vi "TrajectoryBegin.vi"(8 "error in (no error)":errorcluster) -> (0 "error out":errorcluster)   [LabVIEW 2023]
uses:
  TrajectoryGlobals.vi
  <vilib>/Rock Robotics/WPI/ThirdParty/JAS_Junk/TrajLib/Trajectory_Library.lvlib
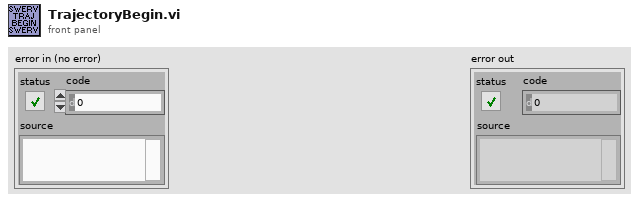
[diagram p1: front panel]
types:
  T1 = typedef "Trajectory_Library.lvlib/TRAJECTORY.ctl" = cluster{"TotalTImeSecs":dbl, "States":T2[]}
  T2 = typedef "Trajectory_Library.lvlib/TRAJ_STATE.ctl" = cluster{"TimeSeconds":dbl, "Velocity":dbl, "Acceleration":dbl, "POSE":T3, "Curvature":dbl}
  T3 = typedef "Trajectory_Library.lvlib/POSE2D.ctl" = cluster{"TRANSLATION":T4, "ROTATION":T5}
  T4 = typedef "Trajectory_Library.lvlib/TRANSLATION2D.ctl" = cluster{"X":dbl, "Y":dbl}
  T5 = typedef "Trajectory_Library.lvlib/ROTATION2D.ctl" = cluster{"VALUE":dbl, "COS":dbl, "SIN":dbl}
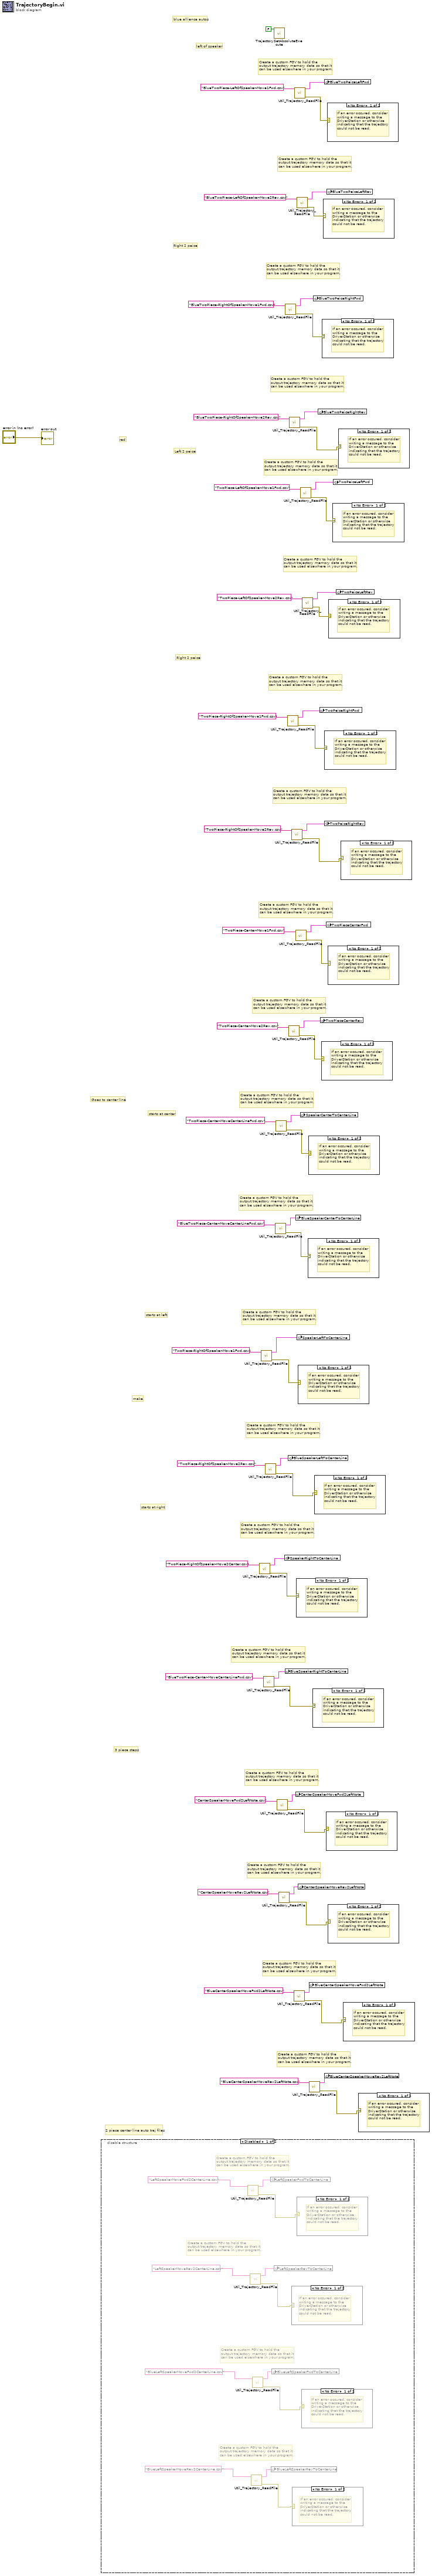
[diagram p0: block diagram]
diagram:
  # "2 piece center line auto traj files"
  # "Create a custom FGV to hold the \noutput trajectory memory data so that it\ncan be used elsewhere in your program."
  # "Create a custom FGV to hold the \noutput trajectory memory data so that it\ncan be used elsewhere in your program."
  # "Create a custom FGV to hold the \noutput trajectory memory data so that it\ncan be used elsewhere in your program."
  # "3 piece steps"
  # "Create a custom FGV to hold the \noutput trajectory memory data so that it\ncan be used elsewhere in your program."
  # "make"
  # "Create a custom FGV to hold the \noutput trajectory memory data so that it\ncan be used elsewhere in your program."
  # "Create a custom FGV to hold the \noutput trajectory memory data so that it\ncan be used elsewhere in your program."
  # "Create a custom FGV to hold the \noutput trajectory memory data so that it\ncan be used elsewhere in your program."
  # "Create a custom FGV to hold the \noutput trajectory memory data so that it\ncan be used elsewhere in your program."
  # "starts at right"
  # "starts at left"
  # "starts at center"
  # "Goes to center line"
  # "Create a custom FGV to hold the \noutput trajectory memory data so that it\ncan be used elsewhere in your program."
  # "Create a custom FGV to hold the \noutput trajectory memory data so that it\ncan be used elsewhere in your program."
  # "Create a custom FGV to hold the \noutput trajectory memory data so that it\ncan be used elsewhere in your program."
  # "Create a custom FGV to hold the \noutput trajectory memory data so that it\ncan be used elsewhere in your program."
  # "red"
  # "Right 2 peice"
  # "Create a custom FGV to hold the \noutput trajectory memory data so that it\ncan be used elsewhere in your program."
  # "Create a custom FGV to hold the \noutput trajectory memory data so that it\ncan be used elsewhere in your program."
  # "Create a custom FGV to hold the \noutput trajectory memory data so that it\ncan be used elsewhere in your program."
  # "Create a custom FGV to hold the \noutput trajectory memory data so that it\ncan be used elsewhere in your program."
  # "left of speaker"
  # "blue allience autos"
  # "Right 2 peice"
  # "Left 2 peice"
  # "Create a custom FGV to hold the \noutput trajectory memory data so that it\ncan be used elsewhere in your program."
  # "Create a custom FGV to hold the \noutput trajectory memory data so that it\ncan be used elsewhere in your program."
  # "Create a custom FGV to hold the \noutput trajectory memory data so that it\ncan be used elsewhere in your program."
  # "Create a custom FGV to hold the \noutput trajectory memory data so that it\ncan be used elsewhere in your program."
  n1 = disable-structure shown="Disabled" {
    frame Disabled {
      # "Create a custom FGV to hold the \noutput trajectory memory data so that it\ncan be used elsewhere in your program."
      # "Create a custom FGV to hold the \noutput trajectory memory data so that it\ncan be used elsewhere in your program."
      # "Create a custom FGV to hold the \noutput trajectory memory data so that it\ncan be used elsewhere in your program."
      # "Create a custom FGV to hold the \noutput trajectory memory data so that it\ncan be used elsewhere in your program."
      n2 = call <vilib>:"Util_Trajectory_ReadFile.vi"("FileName"="LeftSpeakerMoveFwd2CenterLine.csv") -> ("error out"=w72:errorcluster, "outTRAJECTORY"=w73:T1)  [unwired: 8 in, 1 out]
      n3 = call <vilib>:"Util_Trajectory_ReadFile.vi"("FileName"="LeftSpeakerMoveRev2CenterLine.csv") -> ("error out"=w69:errorcluster, "outTRAJECTORY"=w70:T1)  [unwired: 8 in, 1 out]
      n4 = call <vilib>:"Util_Trajectory_ReadFile.vi"("FileName"="BlueLeftSpeakerMoveRev2CenterLine.csv") -> ("error out"=w63:errorcluster, "outTRAJECTORY"=w64:T1)  [unwired: 8 in, 1 out]
      n5 = call <vilib>:"Util_Trajectory_ReadFile.vi"("FileName"="BlueLeftSpeakerMoveFwd2CenterLine.csv") -> ("error out"=w66:errorcluster, "outTRAJECTORY"=w67:T1)  [unwired: 8 in, 1 out]
      n6 = global write "TrajectoryGlobals.vi" "LeftSpeakerFwdToCenterLine"(w73) -> ()
      n7 = global write "TrajectoryGlobals.vi" "BlueLeftSpeakerRevToCenterLine"(w64) -> ()
      n8 = global write "TrajectoryGlobals.vi" "BlueLeftSpeakerFwdToCenterLine"(w67) -> ()
      n9 = global write "TrajectoryGlobals.vi" "LeftSpeakerRevToCenterLine"(w70) -> ()
      n10 = case shown="No Error" w69 {
        frame No Error {
          # "If an error occured, consider\nwriting a message to the\nDriverStation or otherwise\nindicating that the trajectory\ncould not be read."
        }
        frame Error {
        }
      }
      n11 = case shown="No Error" w63 {
        frame No Error {
          # "If an error occured, consider\nwriting a message to the\nDriverStation or otherwise\nindicating that the trajectory\ncould not be read."
        }
        frame Error {
        }
      }
      n12 = case shown="No Error" w72 {
        frame No Error {
          # "If an error occured, consider\nwriting a message to the\nDriverStation or otherwise\nindicating that the trajectory\ncould not be read."
        }
        frame Error {
        }
      }
      n13 = case shown="No Error" w66 {
        frame No Error {
          # "If an error occured, consider\nwriting a message to the\nDriverStation or otherwise\nindicating that the trajectory\ncould not be read."
        }
        frame Error {
        }
      }
    }
    frame Enabled {
    }
  }
  n14 = call <vilib>:"Util_Trajectory_ReadFile.vi"("FileName"="TwoPiece-RightOfSpeaker-Move2Center.csv") -> ("error out"=w23:errorcluster, "outTRAJECTORY"=w24:T1)  [unwired: 8 in, 1 out]
  n15 = call <vilib>:"Util_Trajectory_ReadFile.vi"("FileName"="TwoPiece-RightOfSpeaker-Move1Fwd.csv") -> ("error out"=w17:errorcluster, "outTRAJECTORY"=w18:T1)  [unwired: 8 in, 1 out]
  n16 = call <vilib>:"Util_Trajectory_ReadFile.vi"("FileName"="BlueTwoPiece-Center-MoveCenterLineFwd.csv") -> ("error out"=w20:errorcluster, "outTRAJECTORY"=w21:T1)  [unwired: 8 in, 1 out]
  n17 = call <vilib>:"Util_Trajectory_ReadFile.vi"("FileName"="TwoPiece-RightOfSpeaker-Move2Rev.csv") -> ("error out"=w14:errorcluster, "outTRAJECTORY"=w15:T1)  [unwired: 8 in, 1 out]
  n18 = call "TrajectorySetAbsoluteExecute.vi"("ABSOLUTE EXECUTE"=FALSE) -> ()  [unwired: 11 in]
  n19 = call <vilib>:"Util_Trajectory_ReadFile.vi"("FileName"="BlueTwoPiece-Center-MoveCenterLineFwd.csv") -> ("error out"=w28:errorcluster, "outTRAJECTORY"=w26:T1)  [unwired: 8 in, 1 out]
  n20 = call <vilib>:"Util_Trajectory_ReadFile.vi"("FileName"="TwoPiece-Center-MoveCenterLineFwd.csv") -> ("error out"=w31:errorcluster, "outTRAJECTORY"=w29:T1)  [unwired: 8 in, 1 out]
  n21 = call <vilib>:"Util_Trajectory_ReadFile.vi"("FileName"="CenterSpeakerMoveFwd2LeftNote.csv") -> ("error out"=w11:errorcluster, "outTRAJECTORY"=w12:T1)  [unwired: 8 in, 1 out]
  n22 = call <vilib>:"Util_Trajectory_ReadFile.vi"("FileName"="CenterSpeakerMoveRev2LeftNote.csv") -> ("error out"=w8:errorcluster, "outTRAJECTORY"=w9:T1)  [unwired: 8 in, 1 out]
  n23 = global write "TrajectoryGlobals.vi" "SpeakerRightToCenterLine"(w24) -> ()
  n24 = global write "TrajectoryGlobals.vi" "BlueSpeakerRightToCenterLine"(w21) -> ()
  n25 = call <vilib>:"Util_Trajectory_ReadFile.vi"("FileName"="BlueTwoPiece-RightOfSpeaker-Move1Fwd.csv") -> ("error out"=w41:errorcluster, "outTRAJECTORY"=w42:T1)  [unwired: 8 in, 1 out]
  n26 = call <vilib>:"Util_Trajectory_ReadFile.vi"("FileName"="TwoPiece-RightOfSpeaker-Move1Fwd.csv") -> ("error out"=w53:errorcluster, "outTRAJECTORY"=w54:T1)  [unwired: 8 in, 1 out]
  n27 = global write "TrajectoryGlobals.vi" "BlueSpeakerLeftToCenterLine"(w15) -> ()
  n28 = call <vilib>:"Util_Trajectory_ReadFile.vi"("FileName"="TwoPiece-Center-Move2Rev.csv") -> ("error out"=w34:errorcluster, "outTRAJECTORY"=w32:T1)  [unwired: 8 in, 1 out]
  n29 = call <vilib>:"Util_Trajectory_ReadFile.vi"("FileName"="BlueTwoPiece-RightOfSpeaker-Move2Rev.csv") -> ("error out"=w38:errorcluster, "outTRAJECTORY"=w39:T1)  [unwired: 8 in, 1 out]
  n30 = call <vilib>:"Util_Trajectory_ReadFile.vi"("FileName"="TwoPiece-RightOfSpeaker-Move2Rev.csv") -> ("error out"=w50:errorcluster, "outTRAJECTORY"=w51:T1)  [unwired: 8 in, 1 out]
  n31 = call <vilib>:"Util_Trajectory_ReadFile.vi"("FileName"="BlueCenterSpeakerMoveFwd2LeftNote.csv") -> ("error out"=w5:errorcluster, "outTRAJECTORY"=w6:T1)  [unwired: 8 in, 1 out]
  n32 = call <vilib>:"Util_Trajectory_ReadFile.vi"("FileName"="BlueTwoPiece-LeftOfSpeaker-Move1Fwd.csv") -> ("error out"=w49:errorcluster, "outTRAJECTORY"=w47:T1)  [unwired: 8 in, 1 out]
  n33 = call <vilib>:"Util_Trajectory_ReadFile.vi"("FileName"="TwoPiece-Center-Move1Fwd.csv") -> ("error out"=w37:errorcluster, "outTRAJECTORY"=w35:T1)  [unwired: 8 in, 1 out]
  n34 = global write "TrajectoryGlobals.vi" "CenterSpeakerMoveFwd2LeftNote"(w12) -> ()
  n35 = global write "TrajectoryGlobals.vi" "BlueSpeakerCenterToCenterLine"(w26) -> ()
  n36 = case shown="No Error" w23 {
    frame No Error {
      # "If an error occured, consider\nwriting a message to the\nDriverStation or otherwise\nindicating that the trajectory\ncould not be read."
    }
    frame Error {
    }
  }
  n37 = call <vilib>:"Util_Trajectory_ReadFile.vi"("FileName"="BlueTwoPiece-LeftOfSpeaker-Move2Rev.csv") -> ("error out"=w44:errorcluster, "outTRAJECTORY"=w45:T1)  [unwired: 8 in, 1 out]
  n38 = global write "TrajectoryGlobals.vi" "SpeakerLeftToCenterLine"(w18) -> ()
  n39 = case shown="No Error" w17 {
    frame No Error {
      # "If an error occured, consider\nwriting a message to the\nDriverStation or otherwise\nindicating that the trajectory\ncould not be read."
    }
    frame Error {
    }
  }
  n40 = global write "TrajectoryGlobals.vi" "CenterSpeakerMoveRev2LeftNote"(w9) -> ()
  n41 = call <vilib>:"Util_Trajectory_ReadFile.vi"("FileName"="TwoPiece-LeftOfSpeaker-Move1Fwd.csv") -> ("error out"=w61:errorcluster, "outTRAJECTORY"=w59:T1)  [unwired: 8 in, 1 out]
  n42 = global write "TrajectoryGlobals.vi" "SpeakerCenterToCenterLine"(w29) -> ()
  n43 = call <vilib>:"Util_Trajectory_ReadFile.vi"("FileName"="TwoPiece-LeftOfSpeaker-Move2Rev.csv") -> ("error out"=w56:errorcluster, "outTRAJECTORY"=w57:T1)  [unwired: 8 in, 1 out]
  n44 = case shown="No Error" w28 {
    frame No Error {
      # "If an error occured, consider\nwriting a message to the\nDriverStation or otherwise\nindicating that the trajectory\ncould not be read."
    }
    frame Error {
    }
  }
  n45 = case shown="No Error" w31 {
    frame No Error {
      # "If an error occured, consider\nwriting a message to the\nDriverStation or otherwise\nindicating that the trajectory\ncould not be read."
    }
    frame Error {
    }
  }
  n46 = global write "TrajectoryGlobals.vi" "BlueCenterSpeakerMoveFwd2LeftNote"(w6) -> ()
  n47 = call <vilib>:"Util_Trajectory_ReadFile.vi"("FileName"="BlueCenterSpeakerMoveRev2LeftNote.csv") -> ("error out"=w2:errorcluster, "outTRAJECTORY"=w3:T1)  [unwired: 8 in, 1 out]
  n48 = case shown="No Error" w20 {
    frame No Error {
      # "If an error occured, consider\nwriting a message to the\nDriverStation or otherwise\nindicating that the trajectory\ncould not be read."
    }
    frame Error {
    }
  }
  n49 = global write "TrajectoryGlobals.vi" "BlueTwoPeiceRightFwd"(w42) -> ()
  n50 = case shown="No Error" w14 {
    frame No Error {
      # "If an error occured, consider\nwriting a message to the\nDriverStation or otherwise\nindicating that the trajectory\ncould not be read."
    }
    frame Error {
    }
  }
  n51 = global write "TrajectoryGlobals.vi" "BlueTwoPeiceRightRev"(w39) -> ()
  n52 = global write "TrajectoryGlobals.vi" "TwoPeiceRightFwd"(w54) -> ()
  n53 = global write "TrajectoryGlobals.vi" "TwoPieceCenterRev"(w32) -> ()
  n54 = case shown="No Error" w34 {
    frame No Error {
      # "If an error occured, consider\nwriting a message to the\nDriverStation or otherwise\nindicating that the trajectory\ncould not be read."
    }
    frame Error {
    }
  }
  n55 = case shown="No Error" w41 {
    frame No Error {
      # "If an error occured, consider\nwriting a message to the\nDriverStation or otherwise\nindicating that the trajectory\ncould not be read."
    }
    frame Error {
    }
  }
  n56 = case shown="No Error" w44 {
    frame No Error {
      # "If an error occured, consider\nwriting a message to the\nDriverStation or otherwise\nindicating that the trajectory\ncould not be read."
    }
    frame Error {
    }
  }
  n57 = global write "TrajectoryGlobals.vi" "BlueTwoPeiceLeftFwd"(w47) -> ()
  n58 = global write "TrajectoryGlobals.vi" "TwoPeiceRightRev"(w51) -> ()
  n59 = case shown="No Error" w53 {
    frame No Error {
      # "If an error occured, consider\nwriting a message to the\nDriverStation or otherwise\nindicating that the trajectory\ncould not be read."
    }
    frame Error {
    }
  }
  n60 = global write "TrajectoryGlobals.vi" "BlueCenterSpeakerMoveRev2LeftNote"(w3) -> ()
  n61 = case shown="No Error" w11 {
    frame No Error {
      # "If an error occured, consider\nwriting a message to the\nDriverStation or otherwise\nindicating that the trajectory\ncould not be read."
    }
    frame Error {
    }
  }
  n62 = global write "TrajectoryGlobals.vi" "TwoPieceCenterFwd"(w35) -> ()
  n63 = global write "TrajectoryGlobals.vi" "BlueTwoPeiceLeftRev"(w45) -> ()
  n64 = case shown="No Error" w49 {
    frame No Error {
      # "If an error occured, consider\nwriting a message to the\nDriverStation or otherwise\nindicating that the trajectory\ncould not be read."
    }
    frame Error {
    }
  }
  n65 = case shown="No Error" w37 {
    frame No Error {
      # "If an error occured, consider\nwriting a message to the\nDriverStation or otherwise\nindicating that the trajectory\ncould not be read."
    }
    frame Error {
    }
  }
  n66 = case shown="No Error" w8 {
    frame No Error {
      # "If an error occured, consider\nwriting a message to the\nDriverStation or otherwise\nindicating that the trajectory\ncould not be read."
    }
    frame Error {
    }
  }
  n67 = case shown="No Error" w56 {
    frame No Error {
      # "If an error occured, consider\nwriting a message to the\nDriverStation or otherwise\nindicating that the trajectory\ncould not be read."
    }
    frame Error {
    }
  }
  n68 = case shown="No Error" w61 {
    frame No Error {
      # "If an error occured, consider\nwriting a message to the\nDriverStation or otherwise\nindicating that the trajectory\ncould not be read."
    }
    frame Error {
    }
  }
  n69 = global write "TrajectoryGlobals.vi" "TwoPeiceLeftFwd"(w59) -> ()
  n70 = global write "TrajectoryGlobals.vi" "TwoPeiceLeftRev"(w57) -> ()
  n71 = case shown="No Error" w38 {
    frame No Error {
      # "If an error occured, consider\nwriting a message to the\nDriverStation or otherwise\nindicating that the trajectory\ncould not be read."
    }
    frame Error {
    }
  }
  n72 = case shown="No Error" w50 {
    frame No Error {
      # "If an error occured, consider\nwriting a message to the\nDriverStation or otherwise\nindicating that the trajectory\ncould not be read."
    }
    frame Error {
    }
  }
  n73 = case shown="No Error" w5 {
    frame No Error {
      # "If an error occured, consider\nwriting a message to the\nDriverStation or otherwise\nindicating that the trajectory\ncould not be read."
    }
    frame Error {
    }
  }
  n74 = case shown="No Error" w2 {
    frame No Error {
      # "If an error occured, consider\nwriting a message to the\nDriverStation or otherwise\nindicating that the trajectory\ncould not be read."
    }
    frame Error {
    }
  }
  "error out" <- "error in (no error)"
